vi "Measure_dC_dV.vi"(5 "Junction Name":string, 6 "UiDefinition":T1, 7 ".NET Refnum":refnum<k24>, 8 "new file path (Not A Path if cancelled)":path, 10 "appended path":path, 11 ".NET Refnum in":refnum<k24>) -> (0 "error out":errorcluster, 3 "Cluster":cluster{dbl[], dbl[]})   [LabVIEW 2020]
uses:
  UIReferences.ctl
  D:/LabviewDXFViewer/LabviewDXFViewer/bin/Release/LabviewDXFViewer.exe
  LabviewDXFViewer/bin/Release/LabviewDXFViewer.exe
  <vilib>/Analysis/6fits.llb/Curve Fitting Criteria.ctl
  <vilib>/Utility/file.llb/Write Delimited Spreadsheet (DBL).vi
  <vilib>/Utility/file.llb/Write Delimited Spreadsheet (string).vi
  <vilib>/Analysis/NI_AALPro.lvlib
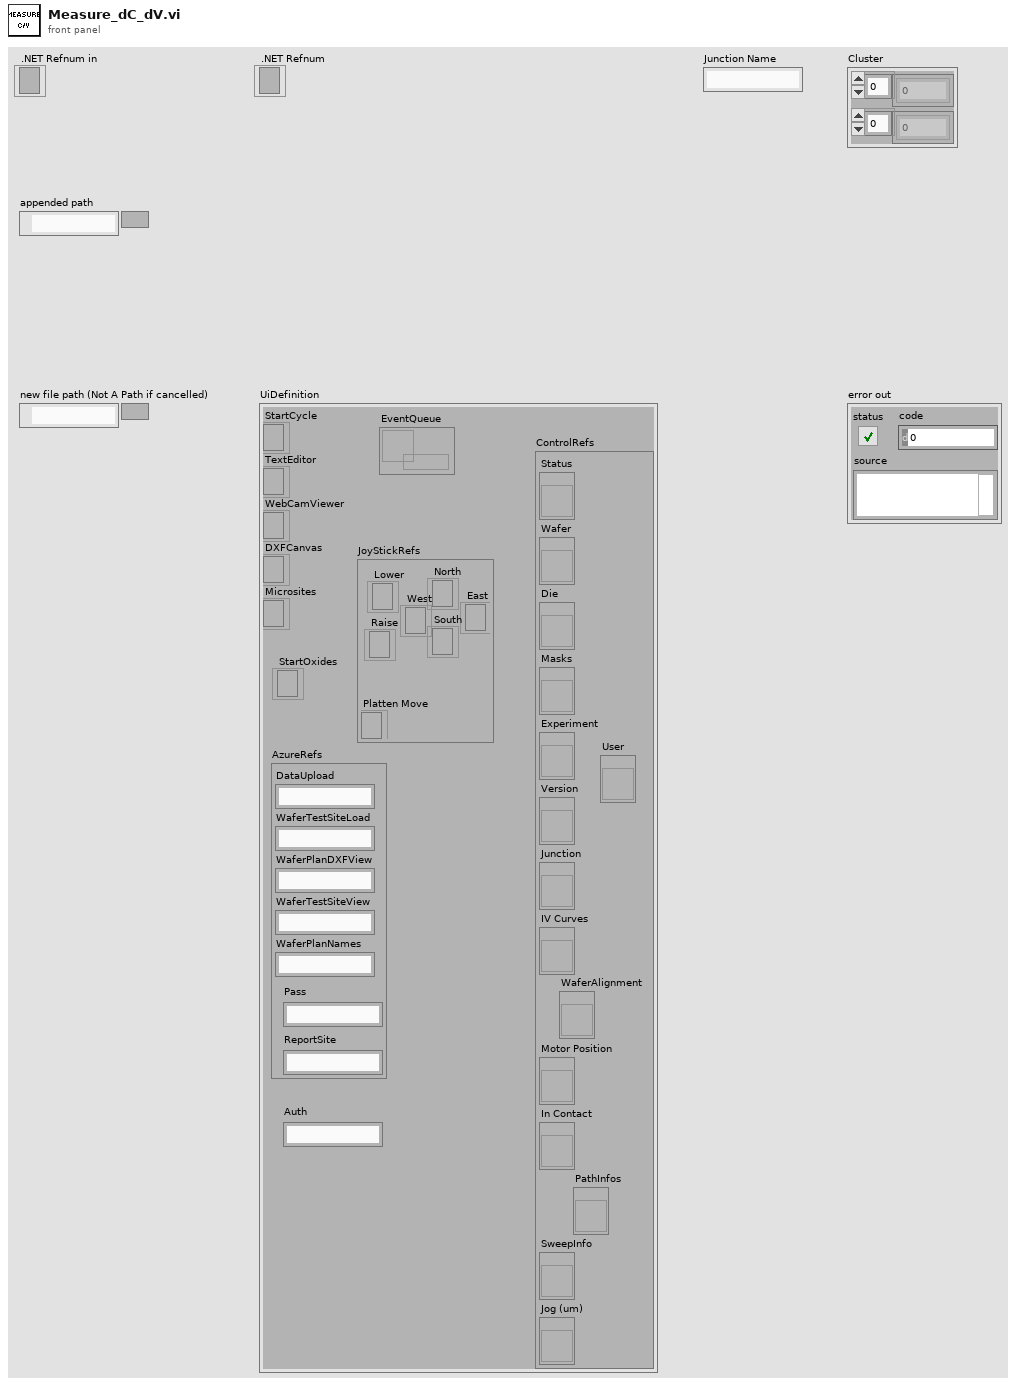
[diagram p1: front panel]
types:
  T1 = typedef "UIReferences.ctl" = cluster{"StartCycle":refnum<k24>, "TextEditor":refnum<k24>, "WebCamViewer":refnum<k24>, "DXFCanvas":refnum<k24>, "Microsites":refnum<k24>, "JoyStickRefs":cluster{"North":refnum<k24>, "Lower":refnum<k24>, "Raise":refnum<k24>, "Platten Move":refnum<k24>, "West":refnum<k24>, "East":refnum<k24>, "South":refnum<k24>}, "AzureRefs":cluster{"DataUpload":string, "WaferTestSiteLoad":string, "WaferPlanDXFView":string, "WaferTestSiteView":string, "WaferPlanNames":string, "Pass":string, "ReportSite":string}, "ControlRefs":cluster{"Status":refnum<vi>, "Wafer":refnum<vi>, "Die":refnum<vi>, "Masks":refnum<vi>, "Experiment":refnum<vi>, "Version":refnum<vi>, "Junction":refnum<vi>, "IV Curves":refnum<vi>, "Motor Position":refnum<vi>, "In Contact":refnum<vi>, "SweepInfo":refnum<vi>, "Jog (um)":refnum<vi>, "PathInfos":refnum<vi>, "User":refnum<vi>, "WaferAlignment":refnum<vi>}, "EventQueue":refnum<queue>, "StartOxides":refnum<k24>, "Auth":string}
  T2 = typedef "NI_AALPro.lvlib/Curve Fitting Criteria.ctl" = u16
  T3 = typedef "CapacitanceInfos.ctl" = cluster{"Conductance":dbl, "CapacitanceIV":dbl, "Intercept":dbl, "CapacitanceSW":dbl, "Sum":dbl, "CapacitanceInfos":T4[], "CapacitancePhase":dbl, "dC/dV":dbl, "Function":string, "OtherInfo":dbl[][]}
  T4 = typedef "CapacitanceRecord.ctl" = cluster{"Freq":dbl, "Vpp":dbl, "PhaseS":dbl, "Irms":dbl, "PhaseC":dbl, "Theta":dbl, "VDrive":dbl, "Capacitance":dbl, "Other":dbl}
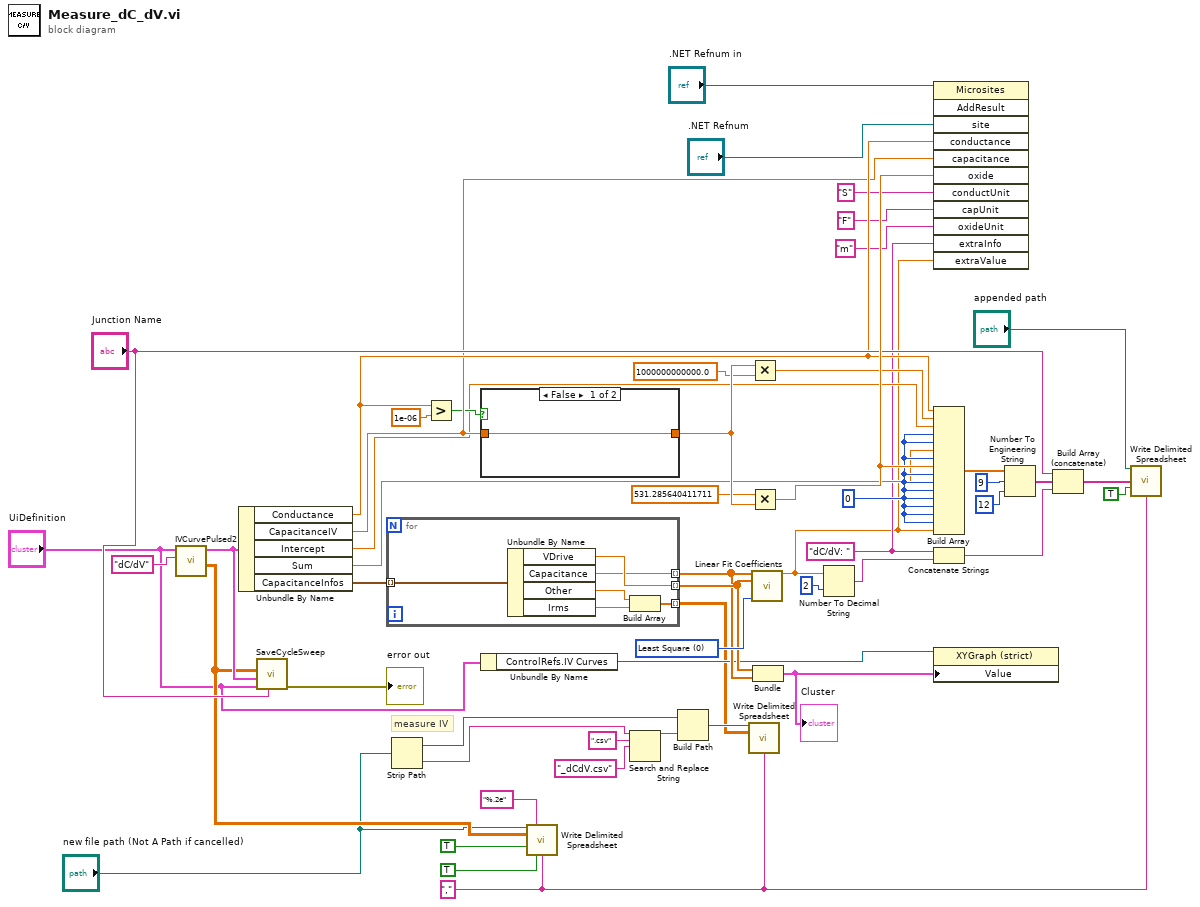
[diagram p0: block diagram]
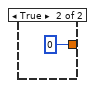
[diagram p2: hidden frame]
diagram:
  w2 = "dC/dV: "
  w7 = "," ("delimiter (\\t)")
  w50 = T2 0 items=["Least Square", "Least Absolute Residual", "Bisquare"] ("method")
  w47 = 0
  # "measure IV"
  n1 = call "IVCurvePulsed2.vi"("Program"="dC/dV", "UiDefinition"="UiDefinition") -> ("appended array"=w26:dbl[][], "InfoCluster"=w39:T3)  [unwired: 8 in]
  n2 = Unbundle By Name(w39) -> ("Conductance"=w41:dbl, "CapacitanceIV"=w40:dbl, "Intercept"=w29:dbl, "Sum"=w30:dbl, "CapacitanceInfos"=w42:T4[])
  n3 = call "SaveCycleSweep.vi"("JunctionName"="Junction Name", "UiDefinition 2"="UiDefinition", "InfoCluster"=w39, "appended array"=w26) -> ("error out"=→"error out":errorcluster)  [unwired: 7 in]
  n4 = for {
    tunnel: w42 -> [w59] mode=indexing
    tunnel: [w58] -> w49 mode=indexing
    tunnel: [w57] -> w48 mode=indexing
    tunnel: [w56] -> w6 mode=indexing
    n5 = Unbundle By Name(w59) -> ("VDrive"=w58:dbl, "Capacitance"=w57:dbl, "Other"=w55:dbl, "Irms"=w54:dbl)
    n6 = Build Array(w55, w54) -> (w56:dbl[])
  }
  n7 = Strip Path(path="new file path (Not A Path if cancelled)") -> (stripped path=w13:path, name=w17:string)
  n8 = Greater?(x=w41, y=1e-06) -> (0:w33:bool)
  n9 = case shown="False" w33 {
    tunnel: [w60 0] -> w52
    tunnel: w40 -> [w60 _]
    frame False {
    }
    frame True {
    }
  }
  n10 = Unbundle By Name("UiDefinition") -> ("ControlRefs.IV Curves"=w12:refnum<vi>)
  n11 = call-poly <vilib>:"Write Delimited Spreadsheet.vi"("file path (dialog if empty)"="new file path (Not A Path if cancelled)", "format (%.3f)"="%.2e", "2D data"=w26, "append to file? (new file:F)"=TRUE, "transpose? (no:F)"=TRUE, "delimiter (\\t)"=w7) -> ()  [unwired: 8 in, 2 out]
  n12 = Search and Replace String(input string=w17, search string=".csv", replace string="_dCdV.csv" ("replace string (\"\")")) -> (result string=w14:string)  [unwired: 5 in, 3 out]
  n13 = Build Path(base path=w13, name or relative path=w14) -> (appended path=w8:path)
  n14 = call-poly <vilib>:"Write Delimited Spreadsheet.vi"("file path (dialog if empty)"=w8, "2D data"=w6, "delimiter (\\t)"=w7) -> ()  [unwired: 11 in, 2 out]
  n15 = Multiply(x=w52, y=1000000000000.0) -> (x*y=w31:dbl)
  n16 = Multiply(x=531.285640411711, y=w52) -> (x*y=w53:dbl)
  n17 = call <vilib>:"Linear Fit Coefficients.vi"("Y"=w48, "X"=w49, "method"=w50) -> ("slope"=w1:dbl)  [unwired: 10 in, 2 out]
  n18 = Bundle(w49, w48) -> (w10:cluster{dbl[], dbl[]})  [unwired: 1 in]
  "Cluster" <- w10
  n19 = Number To Decimal String(number=w1, width (-)=i16 2) -> (decimal integer string=w5:string)
  n20 = invoke class="Microsites" method="AddResult"(reference=".NET Refnum in", "site"=".NET Refnum", "conductance"=w41, "capacitance"=w40, "oxide"=w53, "conductUnit"="S", "capUnit"="F", "oxideUnit"="m" ("interceptUnit"), "extraInfo"=w2, "extraValue"=w1) -> ()  [unwired: 2 in, 12 out]
  n21 = Build Array(w41, w31, w29, w47, w47, w30, w47, w53, w47, w47, w47, w47, w47, w47, w47, w1) -> (w28:dbl[])
  n22 = Concatenate Strings(w2, w5) -> (w3:string)
  n23 = property class="XYGraph (strict)"(reference=w12, "Value"=w10) -> ()  [unwired: 1 in, 2 out]
  n24 = Number To Engineering String(2:i16 12 ("precision (6)"), 3:i16 9 ("width (-)"), 4:w28) -> (0:w20:string[])  [unwired: 1 in]
  n25 = Build Array (concatenate)("Junction Name", w20, w3) -> (w22:string[])
  n26 = call-poly <vilib>:"Write Delimited Spreadsheet.vi"("file path (dialog if empty)"="appended path", "1D data"=w22, "append to file? (new file:F)"=TRUE, "delimiter (\\t)"=w7) -> ()  [unwired: 10 in, 2 out]
